vi "CRYLanguage Check.vi"(11 "sAction":string) -> (2 "Language":T1(ring), 3 "DiffLanguage":bool)   [LabVIEW 2013]
uses:
  CRYMainGlobal.vi
  CRYSystem/Calibration/SubVI/CRYCal Global.vi
  CRYProject/CRYProject Editor Global.vi
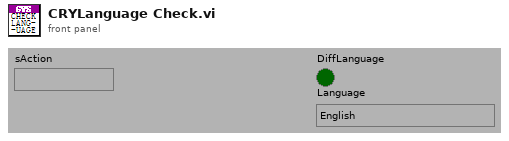
[diagram p1: front panel]
types:
  T1 = enum32{"English", "Chinese", "Korean", "Japanese", "Russian", "Chinese traditional"}
  T2 = typedef "CRYTS.ctl" = cluster{"No.TS":u16, "TS File Path":path, "TS Name":string, "EditStepName":string, "Steps":T3[], "New State":bool, "Change State":bool, "Flattened CurveLib Data":string, "Document Data":string, "EditStepNo":u16, "Operator Start File":string, "Sequence Type":string, "Sequence Language":string}
  T3 = typedef "CRYStep.ctl" = cluster{"No.VI":i32, "Category":string, "StepName":string, "Seq setup flattened":string, "Comment":string, "Steps config.":bool[], "Jump config":i32[], "Start":dbl, "Increment":dbl, "Name":string, "Unit":string, "Y data":u16, "Y prefix":string, "Y dB ref":dbl, "Y unit":string, "Repeat State Array":cluster{"Start":dbl, "Increment":dbl, "Count":i32, "Num":i32}[]}
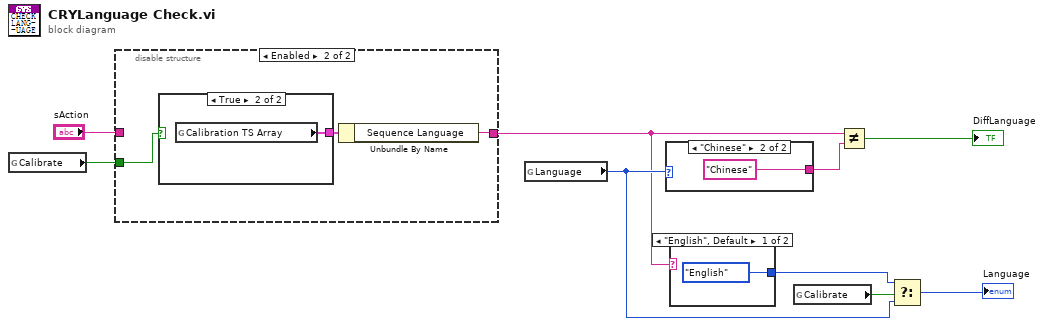
[diagram p0: block diagram]
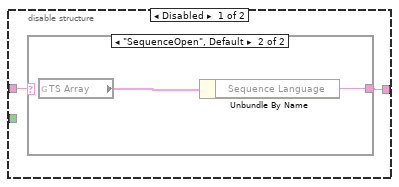
[diagram p2: hidden frame]
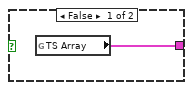
[diagram p4: hidden frame]
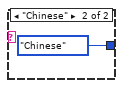
[diagram p5: hidden frame]
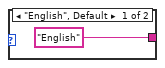
[diagram p6: hidden frame]
diagram:
  n1 = global read "CRYCal Global.vi" "Calibrate"() -> (w1:bool)
  n2 = disable-structure shown="Enabled" {
    disable-tunnel: "sAction" -> [w11 _]
    disable-tunnel: [w10 w16] -> w2
    disable-tunnel: w1 -> [_ w14]
    frame Disabled {
      n3 = case shown="\"SequenceOpen\", Default" w11 {
        tunnel: [_ w12] -> w10
        frame "SequenceInsert" {
        }
        frame "SequenceOpen", Default {
          n4 = global read "CRYProject Editor Global.vi" "TS Array"() -> (w13:T2)
          n5 = Unbundle By Name(w13) -> ("Sequence Language"=w12:string)
        }
      }
    }
    frame Enabled {
      n6 = case shown="True" w14 {
        tunnel: [w17 w18] -> w15
        frame False {
          n7 = global read "CRYProject Editor Global.vi" "TS Array"() -> (w17:T2)
        }
        frame True {
          n8 = global read "CRYProject Editor Global.vi" "Calibration TS Array"() -> (w18:T2)
        }
      }
      n9 = Unbundle By Name(w15) -> ("Sequence Language"=w16:string)
    }
  }
  n10 = global read "CRYMainGlobal.vi" "Language"() -> (w5:T1)
  n11 = case shown="\"Chinese\"" w5 {
    tunnel: ["English" ("TS Name") "Chinese" ("TS Name")] -> w9
    frame "English", Default {
    }
    frame "Chinese" {
    }
  }
  n12 = case shown="\"English\", Default" w2 {
    tunnel: [T1."English" ("Language") T1."Chinese" ("Language")] -> w6
    frame "English", Default {
    }
    frame "Chinese" {
    }
  }
  n13 = global read "CRYCal Global.vi" "Calibrate"() -> (w7:bool)
  n14 = Not Equal?(x=w2, y=w9) -> (x != y?=→"DiffLanguage":bool)
  n15 = Select(t=w6, s=w7, f=w5) -> (s? t:f=→"Language":T1)
